vi "例6-15.vi"() -> ()   [LabVIEW 2019]
uses:
  <vilib>/measure/matone.llb/Harmonic Distortion Analyzer 1 Chan.vi
  <vilib>/Analysis/NI_AALBase.lvlib
  <vilib>/measure/NI_MAPro.lvlib
panel:
  out "谐波幅值":dbl[](array[numeric])
  out "检测的基频值":dbl
  out "THD%":dbl
  in  "谐波次数":dbl=4.0
  in  "采样点数":dbl=1000.0
  in  "采样频率":dbl=1000.0
  in  "基频":dbl=50.0
  out "频谱":T1(graph)
  out "信号波形":waveform(dbl)(graph)
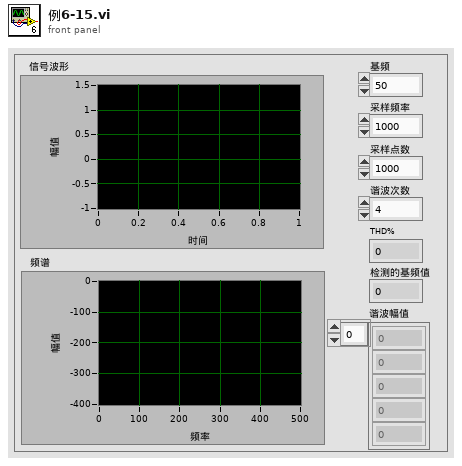
[diagram p1: front panel]
types:
  T1 = cluster{"f0":dbl, "df":dbl, "dB Spectrum (Hann)":dbl[]}
  T2 = enum16{"none", "input signal", "fundamental signal", "residual signal", "harmonics only", "noise and spurs"}
  T3 = cluster{"exported time signal":waveform(dbl), "exported spectrum (dB)":cluster{"f0":dbl, "df":dbl, "dB Spectrum (Hann)":dbl[]}}
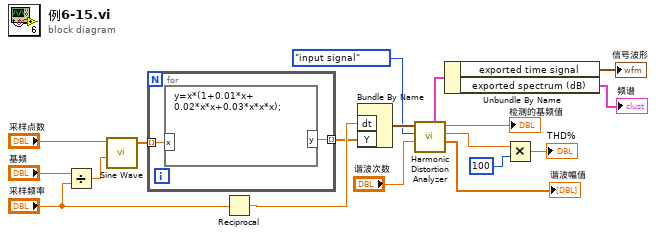
[diagram p0: block diagram]
diagram:
  n1 = Divide(x="基频", y="采样频率") -> (x/y=w16:dbl)
  n2 = call <vilib>:"Sine Wave.vi"("samples"="采样点数", "frequency"=w16) -> ("sine wave"=w15:dbl[])  [unwired: 3 in, 2 out]
  n3 = for {
    tunnel: w15 -> [w20] mode=indexing
    tunnel: [w19] -> w12 mode=indexing
    n4 = formula code="y=x*(1+0.01*x+\n0.02*x*x+0.03*x*x*x);"("x"=w20) -> ("y"=w19:dbl)
  }
  n5 = Reciprocal(x="采样频率") -> (1/x=w13:dbl)
  n6 = Bundle By Name("dt"=w13, "Y"=w12) -> (w11:waveform(dbl))  [unwired: 1 in]
  n7 = call-poly <vilib>:"Harmonic Distortion Analyzer.vi"("highest harmonic"="谐波次数", "export mode"=T2."input signal", "signal in"=w11) -> ("components level"=→"谐波幅值":dbl[], "THD"=w3:dbl, "detected fundamental frequency"=→"检测的基频值":dbl, "exported signals"=w8:T3)  [unwired: 3 in, 2 out]
  n8 = Unbundle By Name(w8) -> ("exported time signal"=→"信号波形":waveform(dbl), "exported spectrum (dB)"=→"频谱":T1)
  n9 = Multiply(x=w3, y=100) -> (x*y=→"THD%":dbl)
